vi "字符串精度转换.vi"(11 "输入字符串":string) -> (3 "输出字符串":string)   [LabVIEW 2016]
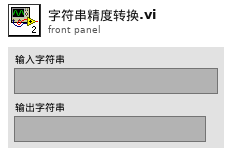
[diagram p1: front panel]
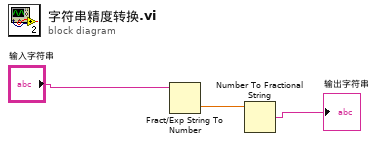
[diagram p0: block diagram]
diagram:
  n1 = Fract/Exp String To Number(string="输入字符串") -> (number=w3:dbl)  [unwired: 3 in, 1 out]
  n2 = Number To Fractional String(number=w3) -> (F-format string=→"输出字符串":string)  [unwired: 3 in]
